vi "Init Before.vi"(11 "Cluster":T1) -> ()   [LabVIEW 2019, in "LSS.lvlib"]
doc: "Intiailize the front panel of the example using property nodes.\n\n<b>Inputs:</b>\n<b>Cluster</b> - Cluster of objects from the front panel of the example."
uses:
  LSS.lvlib
  Before UI References.ctl
  <vilib>/Utility/miscctls.llb/LVBoundsTypeDef.ctl
  <vilib>/Utility/miscctls.llb/LVPositionTypeDef.ctl
  <vilib>/Utility/miscctls.llb/LVPointTypeDef.ctl
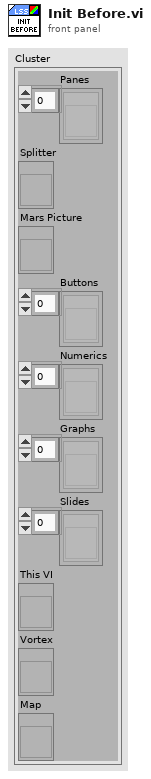
[diagram p1: front panel]
types:
  T1 = typedef "LSS.lvlib/Before UI References.ctl" = cluster{"Panes":refnum<vi>[], "Splitter":refnum<vi>, "Mars Picture":refnum<vi>, "Buttons":refnum<vi>[], "Numerics":refnum<vi>[], "Graphs":refnum<vi>[], "Slides":refnum<vi>[], "This VI":refnum<vi>, "Vortex":refnum<vi>, "Map":refnum<vi>}
  T2 = typedef "LVBoundsTypeDef.ctl" = cluster{"Width":u32, "Height":u32}
  T3 = typedef "LVPositionTypeDef.ctl" = cluster{"Left":i32, "Top":i32}
  T4 = typedef "LVPointTypeDef.ctl" = cluster{"Horizontal":i16, "Vertical":i16}
  T5 = enum16{"Always On", "Always Off", "Off While Running"}
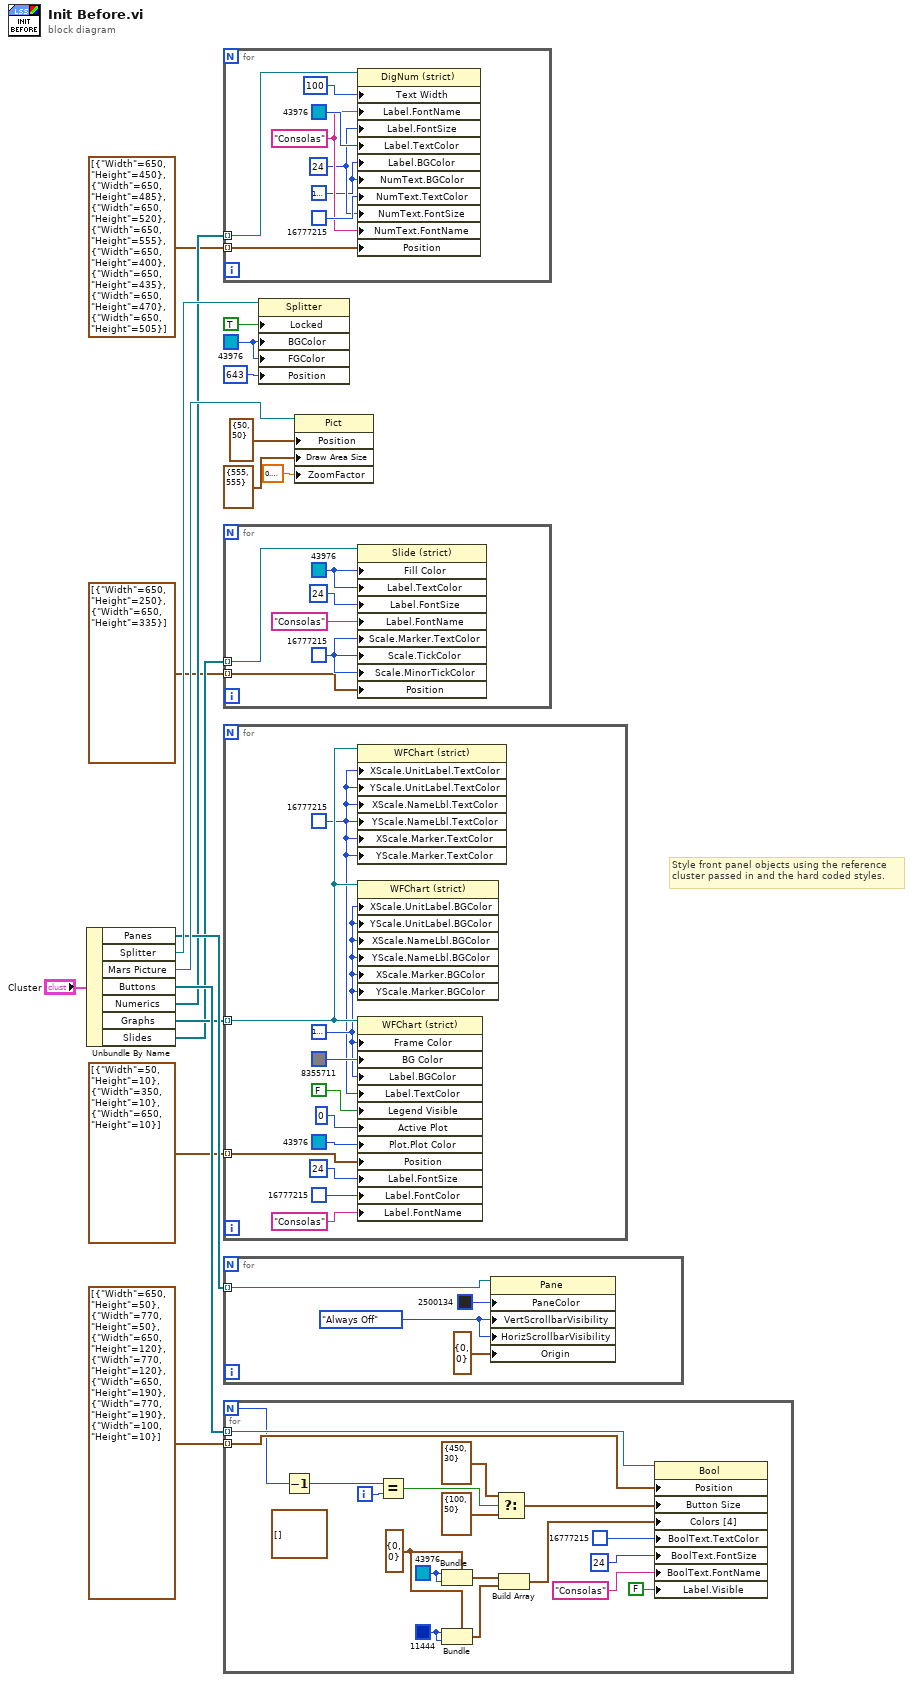
[diagram p0: block diagram]
diagram:
  w9 = u32 43976
  # "Style front panel objects using the reference\ncluster passed in and the hard coded styles."
  n1 = Unbundle By Name("Cluster") -> ("Panes"=w16:refnum<vi>[], "Splitter"=w17:refnum<vi>, "Mars Picture"=w18:refnum<vi>, "Buttons"=w11:refnum<vi>[], "Numerics"=w8:refnum<vi>[], "Graphs"=w6:refnum<vi>[], "Slides"=w5:refnum<vi>[])
  n2 = for {
    tunnel: w8 -> [w26] mode=indexing
    tunnel: T2[] [{"Width"=650, "Height"=450}, {"Width"=650, "Height"=485}, {"Width"=650, "Height"=520}, {"Width"=650, "Height"=555}, {"Width"=650, "Height"=400}, {"Width"=650, "Height"=435}, {"Width"=650, "Height"=470}, {"Width"=650, "Height"=505}] ("Button Size") -> [w19] mode=indexing
    w20 = u32 16777216
    w23 = "Consolas" ("Boolean Text.Font:Name")
    w22 = u32 24 ("Boolean Text.Font:Size")
    n3 = property class="DigNum (strict)"(reference=w26, "Text Width"=u32 100, "Label.FontName"=w23, "Label.FontSize"=w22, "Label.TextColor"=u32 43976, "Label.BGColor"=w20, "NumText.BGColor"=w20, "NumText.TextColor"=u32 16777215, "NumText.FontSize"=w22, "NumText.FontName"=w23, "Position"=w19) -> ()  [unwired: 1 in, 2 out]
  }
  n4 = for {
    tunnel: w5 -> [w32] mode=indexing
    tunnel: T2[] [{"Width"=650, "Height"=250}, {"Width"=650, "Height"=335}] ("Button Size") -> [w27] mode=indexing
    w28 = u32 16777215
    w29 = u32 43976
    n5 = property class="Slide (strict)"(reference=w32, "Fill Color"=w29, "Label.TextColor"=w29, "Label.FontSize"=u32 24 ("Boolean Text.Font:Size"), "Label.FontName"="Consolas" ("Boolean Text.Font:Name"), "Scale.Marker.TextColor"=w28, "Scale.TickColor"=w28, "Scale.MinorTickColor"=w28, "Position"=w27) -> ()  [unwired: 1 in, 2 out]
  }
  n6 = for {
    tunnel: w6 -> [w42] mode=indexing
    tunnel: T2[] [{"Width"=50, "Height"=10}, {"Width"=350, "Height"=10}, {"Width"=650, "Height"=10}] ("Button Size") -> [w36] mode=indexing
    w40 = u32 16777215
    w41 = u32 16777216
    n7 = property class="WFChart (strict)"(reference=w42, "XScale.UnitLabel.TextColor"=w40, "YScale.UnitLabel.TextColor"=w40, "XScale.NameLbl.TextColor"=w40, "YScale.NameLbl.TextColor"=w40, "XScale.Marker.TextColor"=w40, "YScale.Marker.TextColor"=w40) -> ()  [unwired: 1 in, 2 out]
    n8 = property class="WFChart (strict)"(reference=w42, "XScale.UnitLabel.BGColor"=w41, "YScale.UnitLabel.BGColor"=w41, "XScale.NameLbl.BGColor"=w41, "YScale.NameLbl.BGColor"=w41, "XScale.Marker.BGColor"=w41, "YScale.Marker.BGColor"=w41) -> ()  [unwired: 1 in, 2 out]
    n9 = property class="WFChart (strict)"(reference=w42, "Frame Color"=w41, "BG Color"=u32 8355711, "Label.BGColor"=w41, "Label.TextColor"=w40, "Legend Visible"=FALSE ("Legend:Visible"), "Active Plot"=u32 0, "Plot.Plot Color"=u32 43976, "Position"=w36, "Label.FontSize"=u32 24 ("Boolean Text.Font:Size"), "Label.FontColor"=u32 16777215, "Label.FontName"="Consolas" ("Boolean Text.Font:Name")) -> ()  [unwired: 1 in, 2 out]
  }
  n10 = for {
    tunnel: w16 -> [w44] mode=indexing
    w46 = T5."Always Off" ("Vertical Scrollbar Visibility")
    n11 = property on="Property Node" class="Pane"(reference=w44, "PaneColor"=u32 2500134, "VertScrollbarVisibility"=w46, "HorizScrollbarVisibility"=w46, "Origin"=T4 {"Horizontal"=0, "Vertical"=0}) -> ()  [unwired: 1 in, 2 out]
  }
  n12 = for {
    N -> [w54]
    tunnel: w11 -> [w66] mode=indexing
    tunnel: T2[] [{"Width"=650, "Height"=50}, {"Width"=770, "Height"=50}, {"Width"=650, "Height"=120}, {"Width"=770, "Height"=120}, {"Width"=650, "Height"=190}, {"Width"=770, "Height"=190}, {"Width"=100, "Height"=10}] ("Button Size") -> [w60] mode=indexing
    i -> [w52]
    w55 = u32 11444
    w64 = cluster{u32, u32} {0, 0}
    (unwired) cluster{u32, u32}[] [] ("Colors [4]")
    w65 = u32 43976
    n13 = Decrement(x=w54) -> (x-1=w48:i32)
    n14 = Equal?(x=w48, y=w52) -> (x = y?=w53:bool)
    n15 = Bundle(cluster=w64, w65, w65) -> (w63:cluster{u32, u32})
    n16 = Bundle(cluster=w64, w55, w55) -> (w62:cluster{u32, u32})
    n17 = Select(t=T2 {"Width"=450, "Height"=30} ("Button Size"), s=w53, f=T2 {"Width"=100, "Height"=50} ("Button Size")) -> (s? t:f=w49:T2)
    n18 = Build Array(w63, w62) -> (w61:cluster{u32, u32}[])
    n19 = property on="Property Node" class="Bool"(reference=w66, "Position"=w60, "Button Size"=w49, "Colors [4]"=w61, "BoolText.TextColor"=u32 16777215, "BoolText.FontSize"=u32 24 ("Boolean Text.Font:Size"), "BoolText.FontName"="Consolas" ("Boolean Text.Font:Name"), "Label.Visible"=FALSE) -> ()  [unwired: 1 in, 2 out]
  }
  n20 = property on="Property Node" class="Splitter"(reference=w17, "Locked"=TRUE ("Splitter Position Locked"), "BGColor"=w9, "FGColor"=w9, "Position"=643 ("Splitter Position")) -> ()  [unwired: 1 in, 2 out]
  n21 = property on="Property Node" class="Pict"(reference=w18, "Position"=T3 {"Left"=50, "Top"=50}, "Draw Area Size"=T2 {"Width"=555, "Height"=555}, "ZoomFactor"=sgl 0.9 ("Zoom Factor")) -> ()  [unwired: 1 in, 2 out]
